vi "ellipse from parameters.vi"(10 "phi":dbl[](array[numeric]) format="%0.2f", 11 "ellipse parameters":T1) -> (2 "Y":dbl[](array[numeric]), 3 "X":dbl[](array[numeric]))   [LabVIEW 2017]
uses:
  <vilib>/Analysis/coordinate.llb/2D Cartesian Coordinate Rotation (Array).vi
  <vilib>/Analysis/NI_AALPro.lvlib
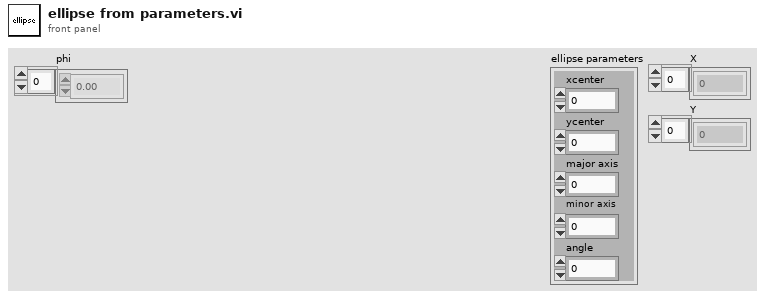
[diagram p1: front panel]
types:
  T1 = cluster{"xcenter":dbl, "ycenter":dbl, "major axis":dbl, "minor axis":dbl, "angle":dbl}
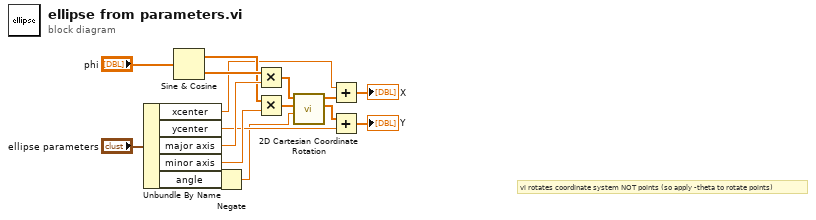
[diagram p0: block diagram]
diagram:
  # "vi rotates coordinate system NOT points (so apply -theta to rotate points)"
  n1 = Unbundle By Name("ellipse parameters") -> ("xcenter"=w8:dbl, "ycenter"=w6:dbl, "major axis"=w14:dbl, "minor axis"=w12:dbl, "angle"=w10:dbl)
  n2 = Sine & Cosine(0:"phi") -> (1:w11:dbl[], 2:w13:dbl[])
  n3 = Negate(x=w10) -> (-x=w1:dbl)
  n4 = Multiply(x=w13, y=w14) -> (x*y=w3:dbl[])
  n5 = Multiply(x=w11, y=w12) -> (x*y=w2:dbl[])
  n6 = call-poly <vilib>:"2D Cartesian Coordinate Rotation.vi"("theta"=w1, "Y"=w2, "X"=w3) -> ("Y Out"=w7:dbl[], "X Out"=w9:dbl[])  [unwired: 6 in, 1 out]
  n7 = Add(x=w8, y=w9) -> (x+y=→"X":dbl[])
  n8 = Add(x=w7, y=w6) -> (x+y=→"Y":dbl[])
